vi "Configure Timebase (Window).vi"(0 "VISA resource name":refnum<visa-resource-name>, 1 "Window Scale (5E-5 s/div)":dbl=5e-05, 5 "Window Position (0.0)":dbl, 9 "Window Range (0.0005 S)":dbl=0.0005, 11 "error in (no error)":errorcluster) -> (4 "VISA resource name out":refnum<visa-resource-name>, 15 "error out":errorcluster)   [LabVIEW 2016, in "Agilent 2000 3000 X-Series.lvlib"]
doc: "Configure the window settings of time base."
uses:
  Agilent 2000 3000 X-Series.lvlib
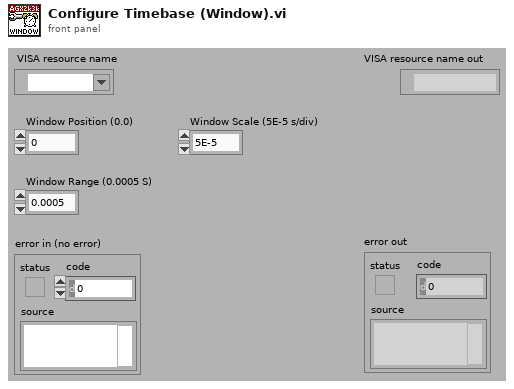
[diagram p1: front panel]
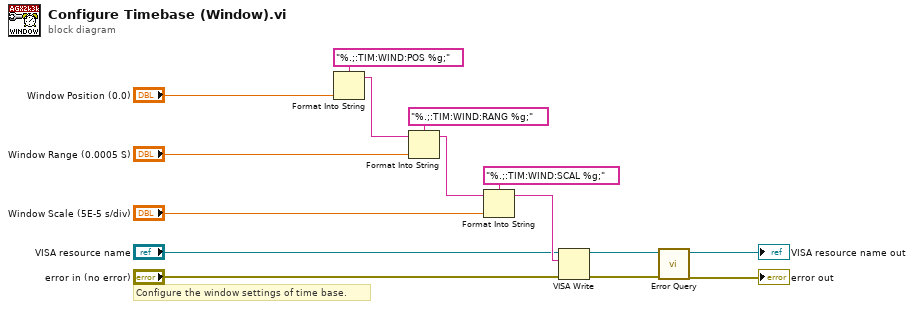
[diagram p0: block diagram]
diagram:
  # "Configure the window settings of time base."
  n1 = Format Into String(format string="%.;:TIM:WIND:POS %g;", "Window Position (0.0)") -> (resulting string=w13:string)  [unwired: 2 in, 1 out]
  n2 = Format Into String(format string="%.;:TIM:WIND:RANG %g;", initial string=w13, "Window Range (0.0005 S)") -> (resulting string=w10:string)  [unwired: 1 in, 1 out]
  n3 = Format Into String(format string="%.;:TIM:WIND:SCAL %g;", initial string=w10, "Window Scale (5E-5 s/div)") -> (resulting string=w7:string)  [unwired: 1 in, 1 out]
  n4 = VISA Write(VISA resource name="VISA resource name", write buffer=w7, error in (no error)="error in (no error)") -> (VISA resource name out=w4:refnum<visa-resource-name>, error out=w3:errorcluster)  [unwired: 1 out]
  n5 = call "Error Query.vi"("error in (no error)"=w3, "VISA resource name"=w4) -> ("error out"=→"error out":errorcluster, "VISA resource name out"=→"VISA resource name out":refnum<visa-resource-name>)  [unwired: 8 out]
